vi "CRYMain Menu Process LIB.vi"(9 "sOption":string, 11 "sAction":string) -> (2 "sData_Out":string)   [LabVIEW 2013]
uses:
  CRYProject/CRYProject Editor Global.vi
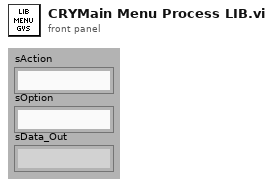
[diagram p1: front panel]
types:
  T1 = enum16{"Left Button", "Center Button", "Right Button", "Window Close"}
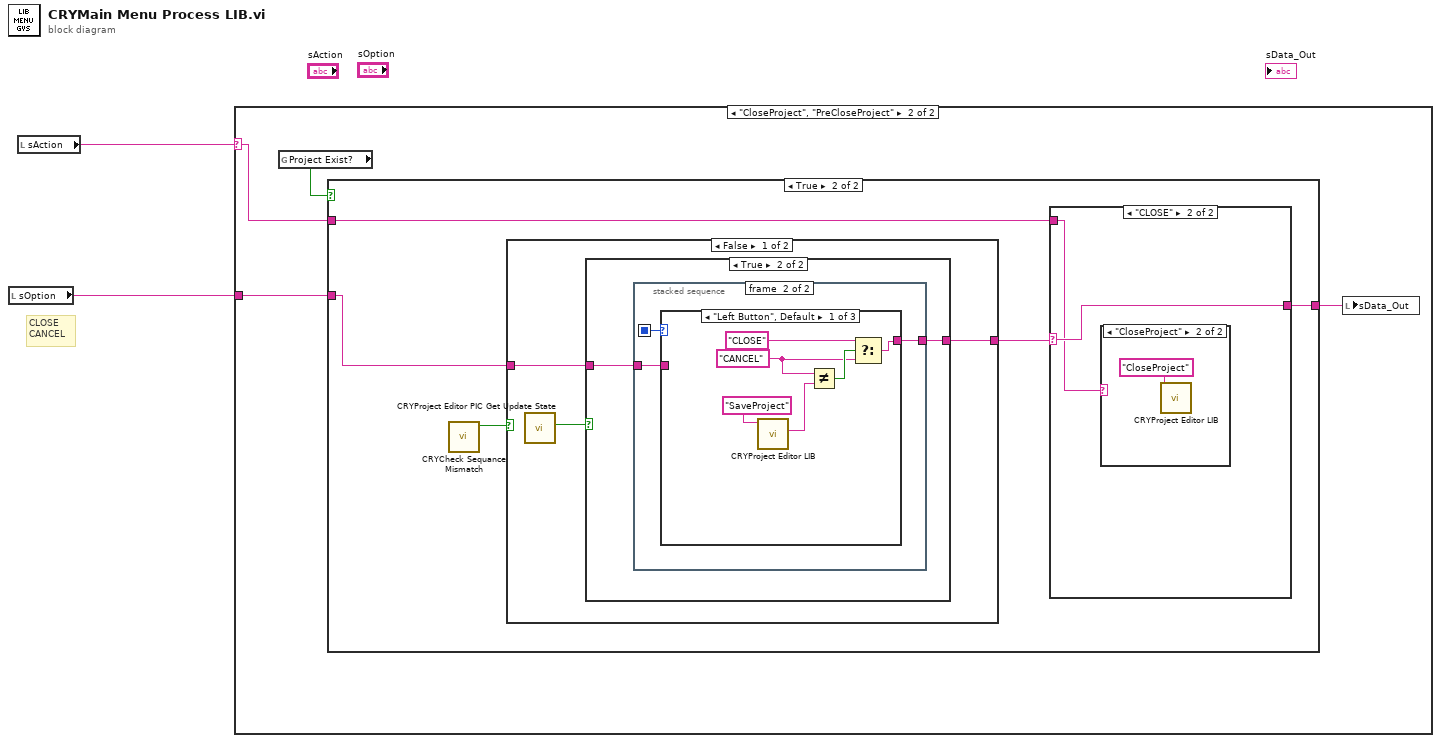
[diagram p0: block diagram]
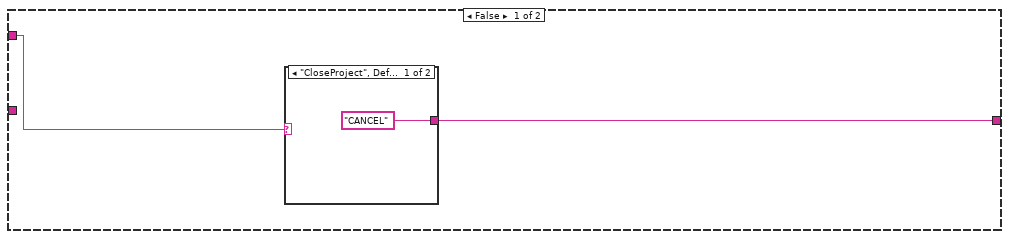
[diagram p3: hidden frame]
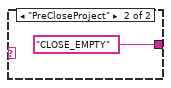
[diagram p4: hidden frame]
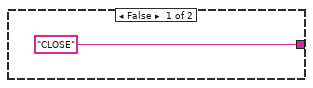
[diagram p5: hidden frame]
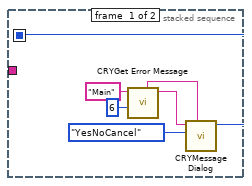
[diagram p6: hidden frame]
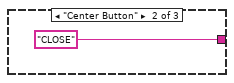
[diagram p7: hidden frame]
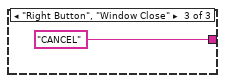
[diagram p8: hidden frame]
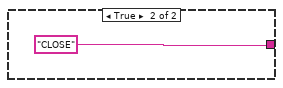
[diagram p9: hidden frame]
diagram:
  # "CLOSE\nCANCEL"
  n1 = local read "sOption"() -> (w1:string)
  n2 = local read "sAction"() -> (w2:string)
  n3 = case shown="\"CloseProject\", \"PreCloseProject\"" w2 {
    selector: w2 -> [_ w3]
    tunnel: w1 -> [_ w5]
    frame "False", Default {
    }
    frame "CloseProject", "PreCloseProject" {
      n4 = global read "CRYProject Editor Global.vi" "Project Exist?"() -> (w6:bool)
      n5 = case shown="True" w6 {
        tunnel: w5 -> [_ w14]
        tunnel: [w8 w13] -> w4
        tunnel: w3 -> [w7 w12]
        frame False {
          n6 = case shown="\"CloseProject\", Default" w7 {
            tunnel: ["CANCEL" "CLOSE_EMPTY"] -> w8
            frame "CloseProject", Default {
            }
            frame "PreCloseProject" {
            }
          }
        }
        frame True {
          n7 = call "CRYCheck Sequance Mismatch.vi"() -> ("Mismatch"=w11:bool)  [unwired: 10 in, 1 out]
          n8 = case shown="False" w11 {
            tunnel: [w18 "CLOSE"] -> w15
            tunnel: w14 -> [w17 _]
            frame False {
              n9 = call "CRYProject Editor PIC Get Update State.vi"() -> ("bChangeState"=w16:bool)  [unwired: 10 in, 1 out]
              n10 = case shown="True" w16 {
                tunnel: ["CLOSE" w21] -> w18
                tunnel: w17 -> [_ w20]
                frame False {
                }
                frame True {
                  n11 = stacked-sequence {
                    seq-local: [w23 _] -> [_ w30]
                    tunnel: [_ w29] -> w21
                    tunnel: w20 -> [_ w28]
                    frame #0 {
                      n12 = call "CRYGet Error Message.vi"("Error No"=6, "Kind"="Main") -> ("Message"=w25:string, "Window Title"=w24:string)  [unwired: 4 in, 4 out]
                      n13 = call "CRYMessage Dialog.vi"("Window Title"=w24, "YesNoCancel"=enum16{"OK", "Yes", "YesNo", "YesNoCancel"}."YesNoCancel", "Message Content"=w25) -> ("Which Button?"=w23:T1)  [unwired: 7 in, 1 out]
                    }
                    frame #1 {
                      n14 = case shown="\"Left Button\", Default" w30 {
                        tunnel: [w35 "CLOSE" "CANCEL"] -> w29
                        tunnel: w28 -> [_ _ _]
                        frame "Left Button", Default {
                          w31 = "CANCEL"
                          n15 = call "CRYProject Editor LIB.vi"("sAction"="SaveProject") -> ("sData_Out"=w34:string)  [unwired: 10 in]
                          n16 = Not Equal?(x=w31, y=w34) -> (x != y?=w33:bool)
                          n17 = Select(t="CLOSE", s=w33, f=w31) -> (s? t:f=w35:string)
                        }
                        frame "Center Button" {
                        }
                        frame "Right Button", "Window Close" {
                        }
                      }
                    }
                  }
                }
              }
            }
            frame True {
            }
          }
          n18 = case shown="\"CLOSE\"" w15 {
            selector: w15 -> [w40 w42]
            tunnel: [w40 w42] -> w13
            tunnel: w12 -> [_ w41]
            frame "CANCEL", Default {
            }
            frame "CLOSE" {
              n19 = case shown="\"CloseProject\"" w41 {
                frame "False", Default {
                }
                frame "CloseProject" {
                  n20 = call "CRYProject Editor LIB.vi"("sAction"="CloseProject") -> ()  [unwired: 10 in, 1 out]
                }
              }
            }
          }
        }
      }
      n21 = local write "sData_Out"(w4) -> ()
    }
  }
